vi "Change_class_Connectors.vi"(11 "vi path":path=path "C:/Users/mrjak/Documents/GitHub/LVGPT/LabVIEW/VIs/Classes/Node") -> ()   [LabVIEW 2025]
uses:
  <vilib>/regexp/Match Regular Expression.xnode
panel:
  out "folder names":string[](array[string])
  out "filenames":string[](array[string])
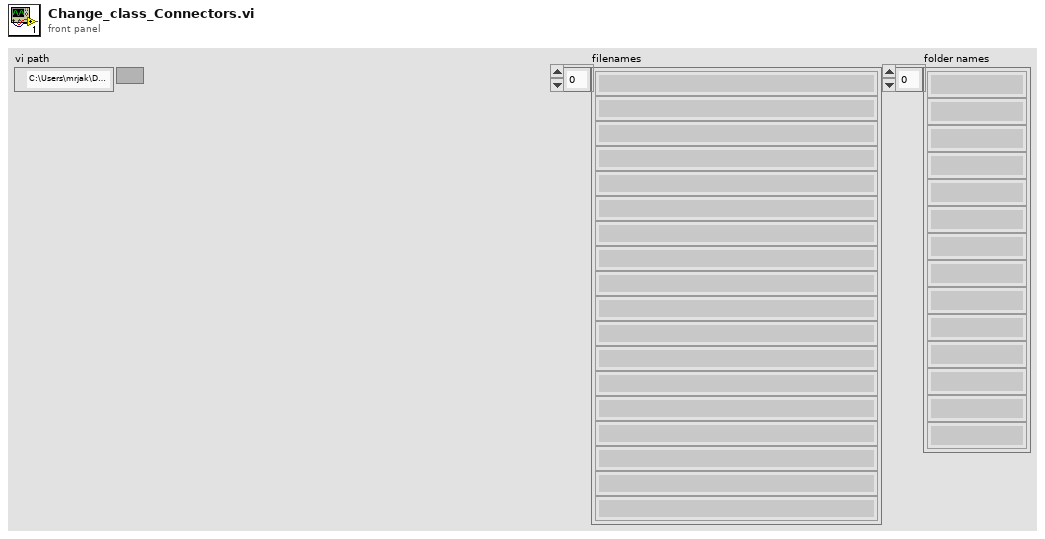
[diagram p1: front panel]
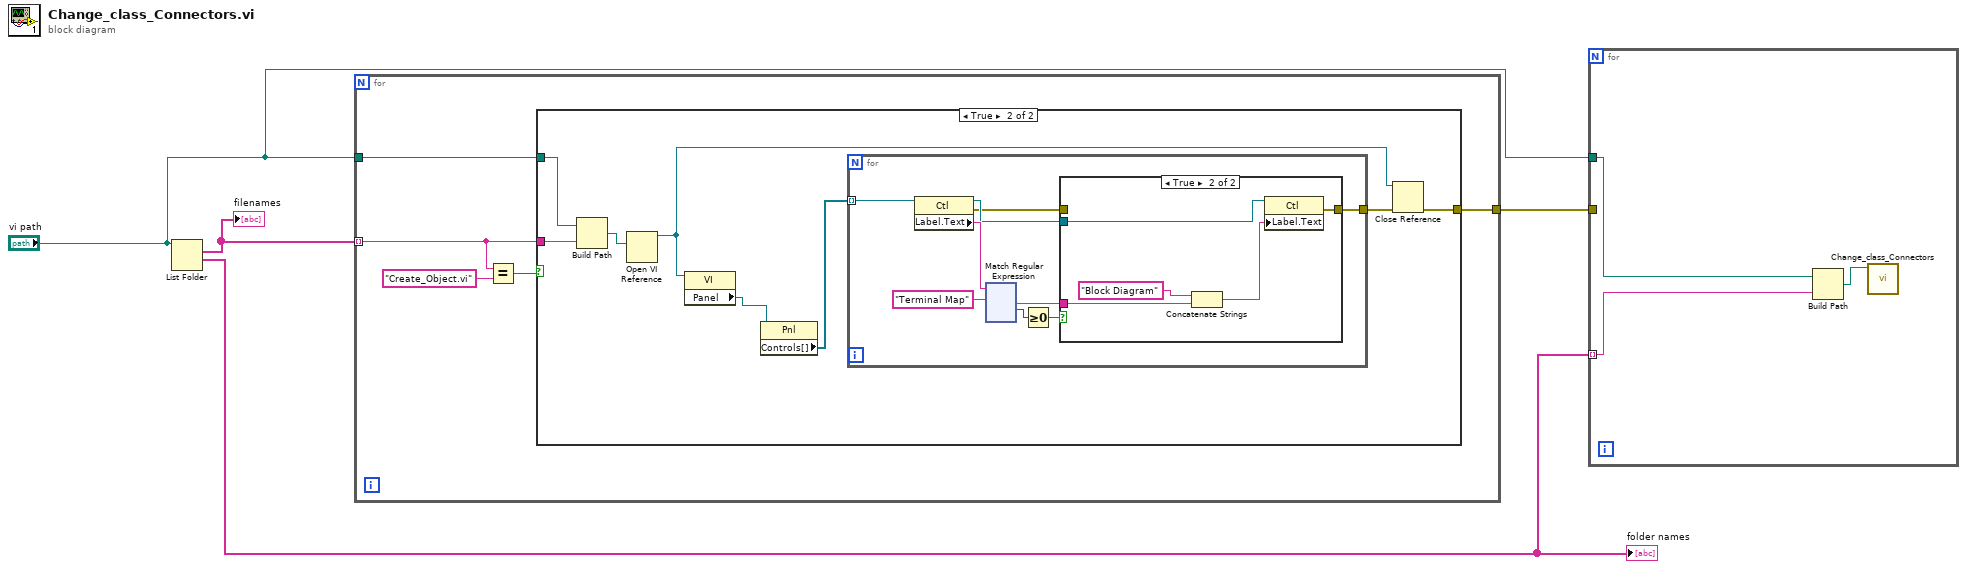
[diagram p0: block diagram]
diagram:
  n1 = List Folder(path="vi path") -> (filenames=w4:string[], folder names=w2:string[])  [unwired: 3 in, 2 out]
  "filenames" <- w4
  "folder names" <- w2
  n2 = for {
    tunnel: "vi path" -> [w9]
    tunnel: w4 -> [w8] mode=indexing
    tunnel: [w5] -> w3
    n3 = Equal?(x=w8, y="Create_Object.vi") -> (x = y?=w7:bool)
    n4 = case shown="True" w7 {
      tunnel: w9 -> [_ w13]
      tunnel: w8 -> [_ w12]
      tunnel: [_ w11] -> w5
      frame False {
      }
      frame True {
        n5 = Build Path(base path=w13, name or relative path=w12) -> (appended path=w10:path)
        n6 = Open VI Reference(vi path=w10) -> (vi reference=w14:refnum<vi>)  [unwired: 5 in, 1 out]
        n7 = property class="VI"(reference=w14) -> ("Panel"=w17:refnum<vi>)  [unwired: 1 in, 2 out]
        n8 = property class="Pnl"(reference=w17) -> ("Controls[]"=w16:refnum<vi>[])  [unwired: 1 in, 2 out]
        n9 = for {
          tunnel: w16 -> [w26] mode=indexing
          tunnel: [w19] -> w15
          n10 = property class="Ctl"(reference=w26) -> (reference out=w21:refnum<vi>, error out=w18:errorcluster, "Label.Text"=w25:string)  [unwired: 1 in]
          n11 = xnode "Match Regular Expression"("input string"=w25, "regular expression"="Terminal Map") -> ("after match"=w20:string, "offset past match"=w23:i32)  [unwired: 4 in, 3 out]
          n12 = Greater Or Equal To 0?(x=w23) -> (x >= 0?=w22:bool)
          n13 = case shown="True" w22 {
            tunnel: w21 -> [_ w32]
            tunnel: w20 -> [_ w30]
            tunnel: [w27 w28] -> w19
            tunnel: w18 -> [w27 _]
            frame False {
            }
            frame True {
              n14 = Concatenate Strings("Block Diagram" ("string"), w30) -> (w29:string)
              n15 = property class="Ctl"(reference=w32, "Label.Text"=w29) -> (error out=w28:errorcluster)  [unwired: 1 in, 1 out]
            }
          }
        }
        n16 = Close Reference(reference=w14, error in (no error)=w15) -> (error out=w11:errorcluster)
      }
    }
  }
  n17 = for {
    tunnel: w3 -> [_]
    tunnel: w2 -> [w150] mode=indexing
    tunnel: "vi path" -> [w151]
    n18 = Build Path(base path=w151, name or relative path=w150) -> (appended path=w152:path)
    n19 = call "Change_class_Connectors.vi"("vi path"=w152) -> ()  [unwired: 11 in]
  }
